vi "IR dat reader.vi"() -> ()   [LabVIEW 2012]
uses:
  <vilib>/Utility/file.llb/Read From Spreadsheet File (I64).vi
panel:
  in  "Stop":bool
  in  "Listbox":i32(listbox)
  out "Waveform Graph":i64[][](graph)
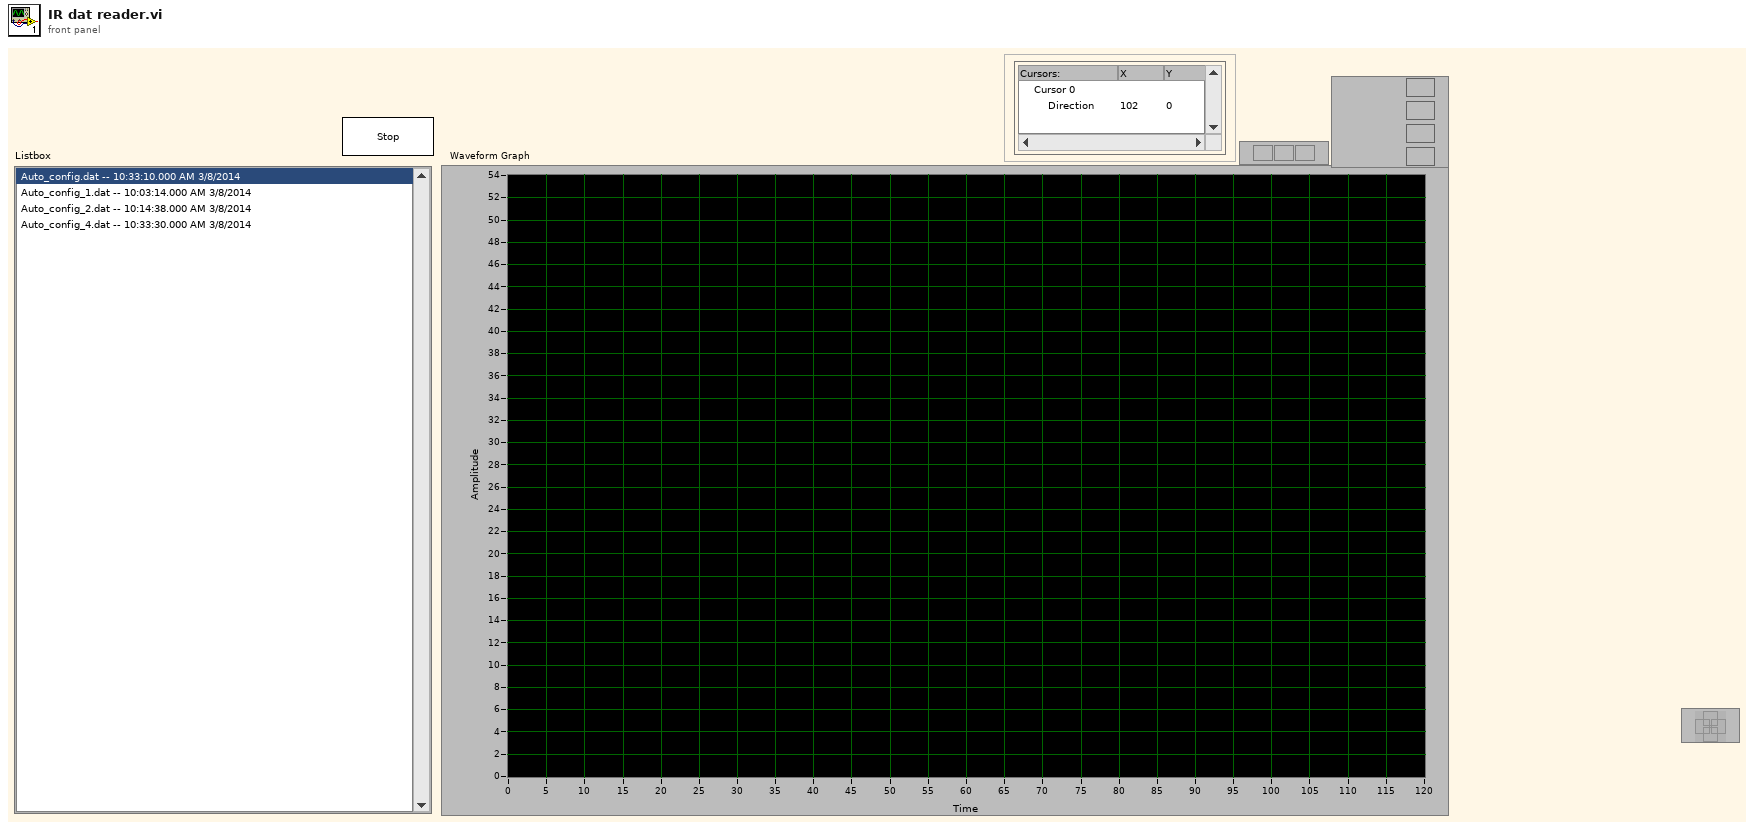
[diagram p1: front panel]
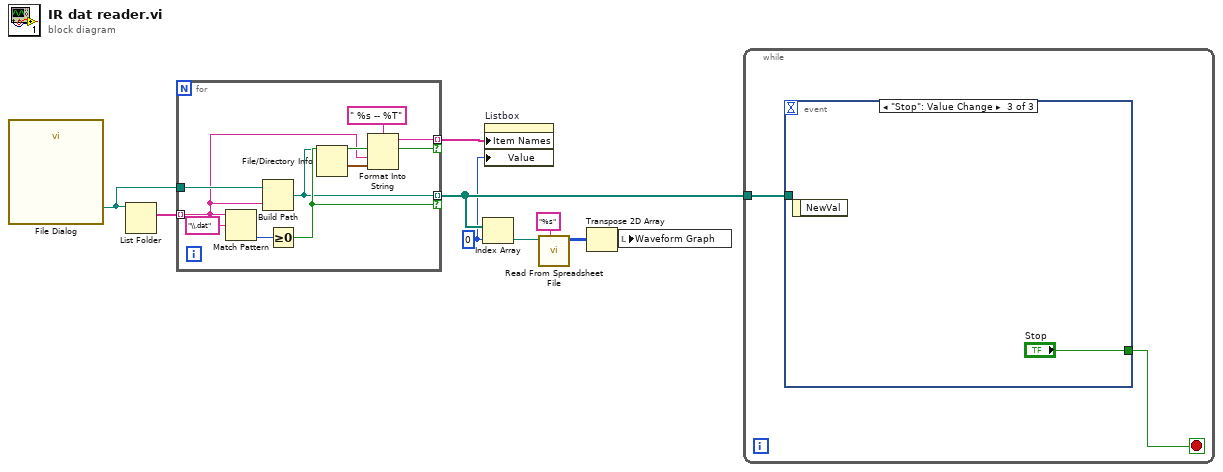
[diagram p0: block diagram]
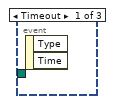
[diagram p2: hidden frame]
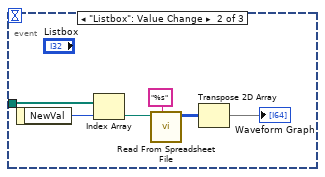
[diagram p3: hidden frame]
diagram:
  w1 = 0 ("index")
  n1 = call "File Dialog"() -> ("selected path"=w8:path)  [unwired: 12 in, 3 out]
  n2 = List Folder(path=w8) -> (filenames=w9:string[])  [unwired: 3 in, 3 out]
  n3 = for {
    tunnel: w9 -> [w12] mode=indexing
    tunnel: w8 -> [w16]
    tunnel: [w10] -> w7 mode=indexing if=w15
    tunnel: [w14] -> w6 mode=indexing if=w15
    n4 = Match Pattern(string=w12, regular expression="\\.dat") -> (offset past match=w17:i32)  [unwired: 1 in, 3 out]
    n5 = Build Path(base path=w16, name or relative path=w12) -> (appended path=w14:path)
    n6 = Greater Or Equal To 0?(x=w17) -> (x >= 0?=w15:bool)
    n7 = File/Directory Info(path=w14) -> (last mod=w13:timestamp)  [unwired: 1 in, 6 out]
    n8 = Format Into String(format string=" %s -- %T", w12, w13) -> (resulting string=w10:string)  [unwired: 2 in, 1 out]
  }
  n9 = Index Array(array=w6, index=w1) -> (element=w3:path)
  n10 = property on="Listbox" class="LstBox (strict)"("Item Names"=w7, "Value"=w1) -> ()  [unwired: 2 in, 2 out]
  n11 = call-poly <vilib>:"Read From Spreadsheet File.vi"("format (%d)"="%s", "file path (dialog if empty)"=w3) -> ("all rows"=w4:i64[][])  [unwired: 5 in, 4 out]
  n12 = Transpose 2D Array(2D array=w4) -> (transposed array=w2:i64[][])
  n13 = local write "Waveform Graph"(w2) -> ()
  n14 = while {
    tunnel: w6 -> [w20]
    stop <- w19 stop-if-true
    n15 = event shown="[2] \"Stop\": Value Change" {
      selector: _ -> [_ _ _]
      dyn-events: _ -> [_ _ _]
      timeout: _ -> [_ _ _]
      tunnel: w20 -> [_ w23 _]
      tunnel: [_ _ "Stop"] -> w19
      event Timeout {
        n16 = event-data() -> ()  [unwired: 1 in, 2 out]
      }
      event "Listbox": Value Change {
        n17 = event-data() -> ("NewVal"=w22:i32)  [unwired: 1 in]
        n18 = Index Array(array=w23, index=w22) -> (element=w21:path)
        n19 = call-poly <vilib>:"Read From Spreadsheet File.vi"("format (%d)"="%s", "file path (dialog if empty)"=w21) -> ("all rows"=w26:i64[][])  [unwired: 5 in, 4 out]
        n20 = Transpose 2D Array(2D array=w26) -> (transposed array=→"Waveform Graph":i64[][])
      }
      event "Stop": Value Change {
        n21 = event-data() -> ()  [unwired: 1 in, 1 out]
      }
    }
  }
